vi "Calc t_0.vi"(8 "error in (no error)":errorcluster, 10 "Sample_Rate_Hz":dbl, 11 "Total_Samples":i64) -> (0 "error out":errorcluster, 3 "t_0":timestamp)   [LabVIEW 2026, in "Acquisition.lvlib"]
uses:
  Acquisition.lvlib
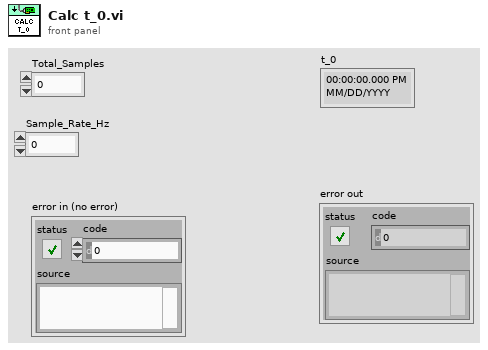
[diagram p1: front panel]
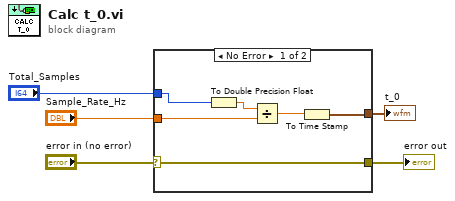
[diagram p0: block diagram]
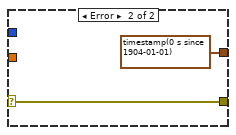
[diagram p2: hidden frame]
diagram:
  n1 = case shown="No Error" "error in (no error)" {
    selector: "error in (no error)" -> [w11 w13]
    tunnel: [w11 w13] -> w4
    tunnel: "Total_Samples" -> [w9 _]
    tunnel: "Sample_Rate_Hz" -> [w10 _]
    tunnel: [w6 timestamp(0 s since 1904-01-01)] -> w1
    frame No Error {
      n2 = To Double Precision Float(number=w9) -> (double precision float=w8:dbl)
      n3 = Divide(x=w8, y=w10) -> (x/y=w7:dbl)
      n4 = To Time Stamp(1:w7) -> (0:w6:timestamp)
    }
    frame Error {
    }
  }
  "error out" <- w4
  "t_0" <- w1
